vi "signal_analysis.vi"() -> ()   [LabVIEW 2018]
panel:
  in  "Dial":dbl(knob) scale=0.0..10.0
  in  "stop":bool
  out "Frequency":dbl
  out "Amplitude":dbl
  out "Waveform Chart":dynamicdata(graph)
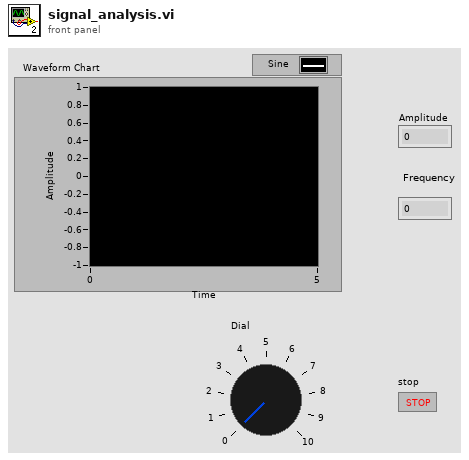
[diagram p1: front panel]
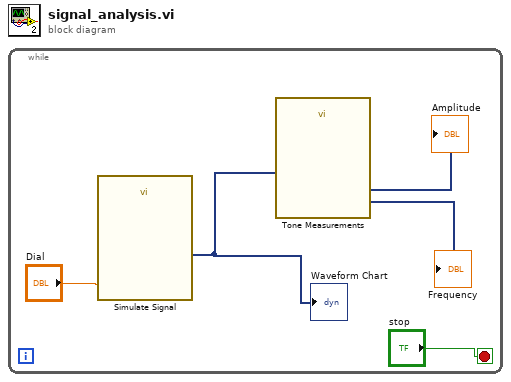
[diagram p0: block diagram]
diagram:
  n1 = while {
    stop <- "stop" stop-if-true
    n2 = call "Simulate Signal"("Frequency"="Dial") -> ("Sine"=w1:dynamicdata)  [unwired: 13 in, 1 out]
    "Waveform Chart" <- w1
    n3 = call "Tone Measurements"("Signals"=w1) -> ("Frequency"=→"Frequency":dynamicdata, "Amplitude"=→"Amplitude":dynamicdata)  [unwired: 8 in, 1 out]
  }
